vi "Tag to Component.vi"(11 "Item Tag in":string) -> (2 "Component Value":string, 3 "Component Name":string)   [LabVIEW 2016, in "Assert API Components.lvlib" / "Assert Display.lvlib" / "Main Display.lvlib" / "RCM_Actions.lvclass"]
uses:
  RCM_Actions.lvclass
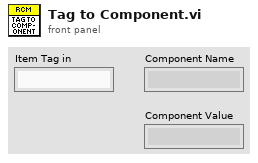
[diagram p1: front panel]
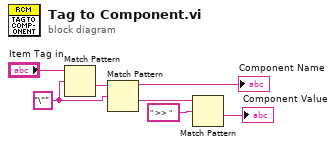
[diagram p0: block diagram]
diagram:
  w2 = "\"" ("regular expression")
  n1 = Match Pattern(string="Item Tag in", regular expression=w2) -> (after substring=w1:string)  [unwired: 1 in, 3 out]
  n2 = Match Pattern(string=w1, regular expression=w2) -> (before substring=→"Component Name":string, after substring=w3:string)  [unwired: 1 in, 2 out]
  n3 = Match Pattern(string=w3, regular expression=" >> ") -> (after substring=→"Component Value":string)  [unwired: 1 in, 3 out]
